vi "GEN_FrontPanel Delay.vi"(7 "VI ref":refnum<vi>, 9 "错误输入（无错误）":errorcluster, 10 "delay？":bool) -> (1 "错误输出":errorcluster)   [LabVIEW 2016]
doc: "设置前面板延时更新的属性\n第一次执行时需要输入VI Ref端"
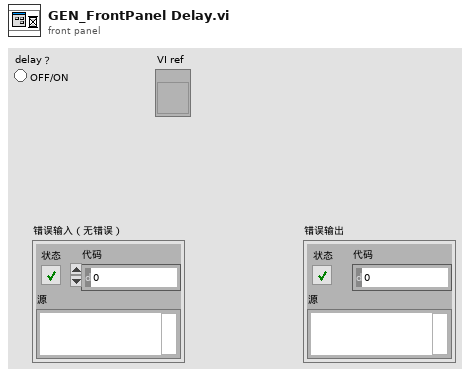
[diagram p1: front panel]
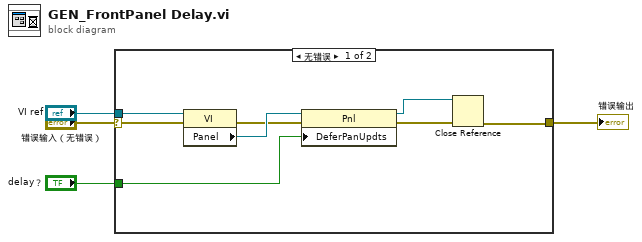
[diagram p0: block diagram]
diagram:
  n1 = case shown="无错误" "错误输入（无错误）" {
    selector: "错误输入（无错误）" -> [w11 w13]
    tunnel: "VI ref" -> [w10 _]
    tunnel: "delay？" -> [w12 _]
    tunnel: [w5 w13] -> w2
    frame No Error {
      n2 = property class="VI"(reference=w10, error in=w11) -> (error out=w8:errorcluster, "Panel"=w9:refnum<vi>)  [unwired: 1 out]
      n3 = property class="Pnl"(reference=w9, error in=w8, "DeferPanUpdts"=w12) -> (reference out=w6:refnum<vi>, error out=w7:errorcluster)
      n4 = Close Reference(reference=w6, error in (no error)=w7) -> (error out=w5:errorcluster)
    }
    frame Error {
    }
  }
  "错误输出" <- w2
